vi "Get MW-HR Limits.vi"(8 "error in (no error)":errorcluster, 11 "Cell":string) -> (0 "error out":errorcluster, 1 "Max MW-HR":dbl format="%.2f", 2 "MW-HR Remain":dbl format="%.2f")   [LabVIEW 2020]
uses:
  <vilib>/Utility/config.llb/Read Key (Double).vi
  <vilib>/Utility/config.llb/NI_LVConfig.lvlib
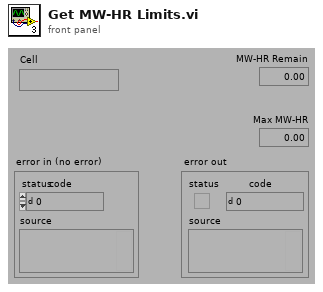
[diagram p1: front panel]
types:
  T1 = typedef "NI_LVConfig.lvlib/Config Data RefNum.ctl" = refnum<k1>
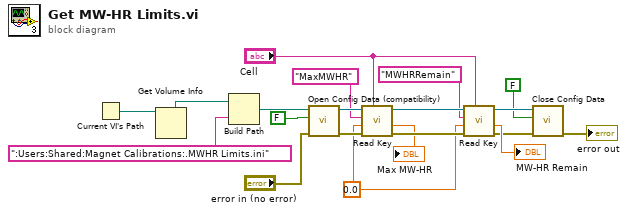
[diagram p0: block diagram]
diagram:
  w16 = 0.0
  n1 = Current VI's Path() -> (path=w15:path)
  n2 = Get Volume Info(11:w15) -> (5:w13:path)  [unwired: 1 in, 5 out]
  n3 = Build Path(base path=w13, name or relative path=":Users:Shared:Magnet Calibrations:.MWHR Limits.ini") -> (appended path=w12:path)
  n4 = call <vilib>:"Open Config Data (compatibility).vi"("error in (no error)"="error in (no error)", "create file if necessary (T)"=FALSE ("create file if necessary? (T)"), "configuration file path"=w12) -> ("error out"=w20:errorcluster, "refnum"=w19:T1)  [unwired: 6 in, 1 out]
  n5 = call-poly <vilib>:"Read Key.vi"("section"="Cell", "error in (no error)"=w20, "default value"=w16, "key"="MaxMWHR", "refnum"=w19) -> ("error out"=w18:errorcluster, "value"=→"Max MW-HR":dbl, "refnum out"=w17:T1)  [unwired: 3 in, 1 out]
  n6 = call-poly <vilib>:"Read Key.vi"("section"="Cell", "error in (no error)"=w18, "default value"=w16, "key"="MWHRRemain", "refnum"=w17) -> ("error out"=w4:errorcluster, "value"=→"MW-HR Remain":dbl, "refnum out"=w3:T1)  [unwired: 3 in, 1 out]
  n7 = call <vilib>:"Close Config Data.vi"("error in (no error)"=w4, "write file if changed (T)"=FALSE ("write configuration file? (T)"), "refnum"=w3) -> ("error out"=→"error out":errorcluster)  [unwired: 7 in, 1 out]
